vi "Pose2d_Div.vi"(9 "Scalar":dbl, 11 "in POSE":T1 {"ROTATION"."SIN" format="%13.4f"; "ROTATION"."COS" format="%13.4f"; "ROTATION"."VALUE" format="%13.4f"; "TRANSLATION"."Y" format="%14.3f"; "TRANSLATION"."X" format="%14.3f"}) -> (3 "out POSE":T1 {"ROTATION"."SIN" format="%13.4f"; "ROTATION"."COS" format="%13.4f"; "ROTATION"."VALUE" format="%13.4f"; "TRANSLATION"."Y" format="%14.3f"; "TRANSLATION"."X" format="%14.3f"})   [LabVIEW 2019, in "Trajectory_Library.lvlib"]
doc: "Divide the pose by the given scalar\"\n\n\nParameters:\n - IN POSE - The input POSE data structure\n - Scalar - The value to divide the pose by.\n\nReturn:\n - OUT POSE - The output pose."
uses:
  TypeDef/POSE2D.ctl
  TypeDef/TRANSLATION2D.ctl
  TypeDef/ROTATION2D.ctl
  Translation2d_Create.vi
  Rotation2d_CreateAngle.vi
  Trajectory_Library.lvlib
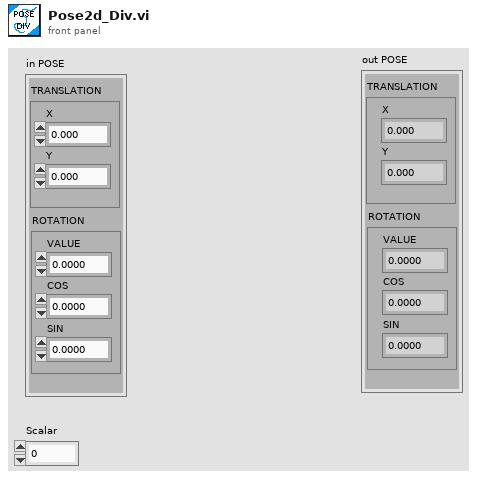
[diagram p1: front panel]
types:
  T1 = typedef "Trajectory_Library.lvlib/POSE2D.ctl" = cluster{"TRANSLATION":T2, "ROTATION":T3}
  T2 = typedef "Trajectory_Library.lvlib/TRANSLATION2D.ctl" = cluster{"X":dbl, "Y":dbl}
  T3 = typedef "Trajectory_Library.lvlib/ROTATION2D.ctl" = cluster{"VALUE":dbl, "COS":dbl, "SIN":dbl}
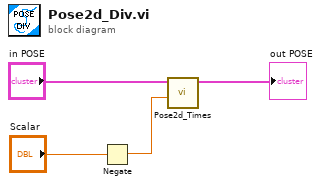
[diagram p0: block diagram]
diagram:
  n1 = Negate(x="Scalar") -> (-x=w3:dbl)
  n2 = call "Pose2d_Times.vi"("Scalar"=w3, "in POSE"="in POSE") -> ("out POSE"=→"out POSE":T1)  [unwired: 9 in]
